vi "writeScanObj.vi"(4 "error in":errorcluster, 5 "OCT filename in":string, 6 "Output Path":path=path "E:/test", 7 "Scan":refnum<class "Scan.lvclass">) -> (0 "error out":errorcluster, 2 "ScanObj ffname":path, 3 "Scan out":refnum<class "Scan.lvclass">)   [LabVIEW 2017]
uses:
  classes/Scans/Scan.lvclass
panel:
  in  "replace string (\"\")":string="-scanobj"
  in  "search string":string=".octa"
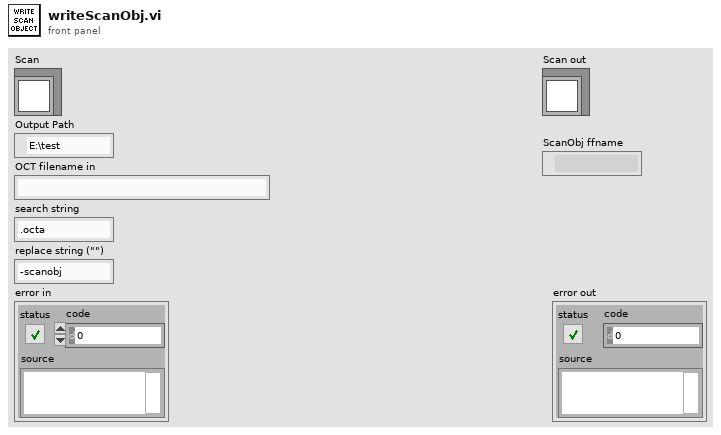
[diagram p1: front panel]
types:
  T1 = enum16{"open", "replace", "create", "open or create", "replace or create", "replace or create with confirmation"}
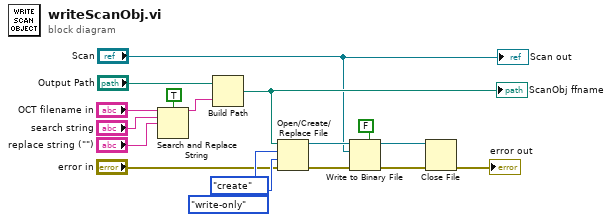
[diagram p0: block diagram]
diagram:
  n1 = Search and Replace String(case sensitive?=TRUE ("ignore case? (F)"), input string="OCT filename in", search string="search string", replace string="replace string (\"\")") -> (result string=w1:string)  [unwired: 4 in, 3 out]
  n2 = Build Path(base path="Output Path", name or relative path=w1) -> (appended path=w7:path)
  "ScanObj ffname" <- w7
  n3 = Open/Create/Replace File(file path (use dialog)=w7, error in="error in", operation (0:open)=T1."create", access (0:read/write)=enum16{"read/write", "read-only", "write-only"}."write-only") -> (refnum out=w11:refnum<file>, error out=w12:errorcluster)  [unwired: 2 in, 1 out]
  n4 = Write to Binary File(file (use dialog)=w11, data="Scan", error in=w12, 5:FALSE ("prepend array or string size? (T)")) -> (refnum out=w9:refnum<file>, error out=w10:errorcluster)  [unwired: 2 in, 1 out]
  n5 = Close File(refnum=w9, error in=w10) -> (error out=→"error out":errorcluster)  [unwired: 1 out]
  "Scan out" <- "Scan"
